vi "KeyboardControl2_PC_Main.vi"() -> ()   [LabVIEW 2014]
uses:
  <vilib>/Utility/inputDevices.llb/keyboardAcquire.vi
  <vilib>/Utility/inputDevices.llb/closeKeyboard.vi
panel:
  in  "Control Selector":bool
  in  "stop":bool
  out "ServoKeyboard":dbl min=-45.0 max=45.0 step=1.0
  out "PropmotorKeybd":dbl min=-9.0 max=9.0 step=1.0
  out "RT Blink":bool
  out "error IO":errorcluster
  out "PC running":bool
  # "Potentiometer"
  # "Use the arrow keys and the \"/\"\nthe change the values"
  # "Keyboard"
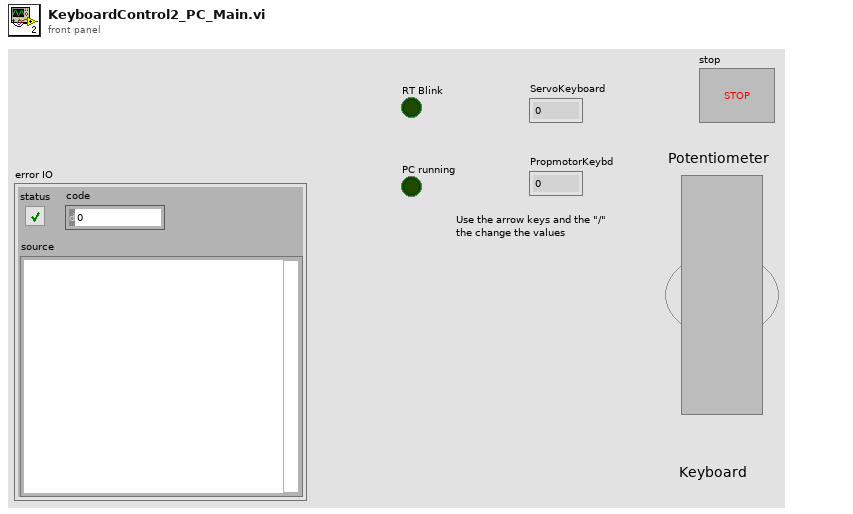
[diagram p1: front panel]
types:
  T1 = enum16{"0", "1", "2", "3", "4", "5", "6", "7", "8", "9", "A", "B", "C", "D", "E", "F", "G", "H", "I", "J", "K", "L", "M", "N", "O", "P", "Q", "R", "S", "T", "U", "V", "W", "X", "Y", "Z", "F1", "F2", "F3", "F4", "F5", "F6", "F7", "F8", "F9", "F10", "F11", "F12", "F13", "F14", "F15", "ADD", "BACK", "BACKSLASH", "CAPITAL", "COMMA", "DECIMAL", "DELETE", "DIVIDE", "DOWN", "END", "EQUALS", "ESCAPE", "GRAVE (`)", "HOME", "INSERT", "LBRACKET", "LCONTROL", "LEFT", "L ALT", "LSHIFT", "LWIN", "MINUS", "MULTIPLY", "NEXT", "NUMLOCK", "NUMPAD_0", "NUMPAD_1", "NUMPAD_2", "NUMPAD_3", "NUMPAD_4", "NUMPAD_5", "NUMPAD_6", "NUMPAD_7", "NUMPAD_8", "NUMPAD_9", "PAUSE", "PERIOD", "PRIOR (PG UP)", "RBRACKET", "RCONTROL", "RETURN", "RIGHT", "R ALT", "RSHIFT", "RWIN", "SCROLL", "SEMICOLON", "SLASH", "SPACE", "SUBTRACT", "TAB", "UP", "ENTER (num pad)", "' (quote)"}[]
  T2 = enum16{"0", "1", "2", "3", "4", "5", "6", "7", "8", "9", "A", "B", "C", "D", "E", "F", "G", "H", "I", "J", "K", "L", "M", "N", "O", "P", "Q", "R", "S", "T", "U", "V", "W", "X", "Y", "Z", "F1", "F2", "F3", "F4", "F5", "F6", "F7", "F8", "F9", "F10", "F11", "F12", "F13", "F14", "F15", "ADD", "BACK", "BACKSLASH", "CAPITAL", "COMMA", "DECIMAL", "DELETE", "DIVIDE", "DOWN", "END", "EQUALS", "ESCAPE", "GRAVE (`)", "HOME", "INSERT", "LBRACKET", "LCONTROL", "LEFT", "L ALT", "LSHIFT", "LWIN", "MINUS", "MULTIPLY", "NEXT", "NUMLOCK", "NUMPAD_0", "NUMPAD_1", "NUMPAD_2", "NUMPAD_3", "NUMPAD_4", "NUMPAD_5", "NUMPAD_6", "NUMPAD_7", "NUMPAD_8", "NUMPAD_9", "PAUSE", "PERIOD", "PRIOR (PG UP)", "RBRACKET", "RCONTROL", "RETURN", "RIGHT", "R ALT", "RSHIFT", "RWIN", "SCROLL", "SEMICOLON", "SLASH", "SPACE", "SUBTRACT", "TAB", "UP", "ENTER (num pad)", "' (quote)"}
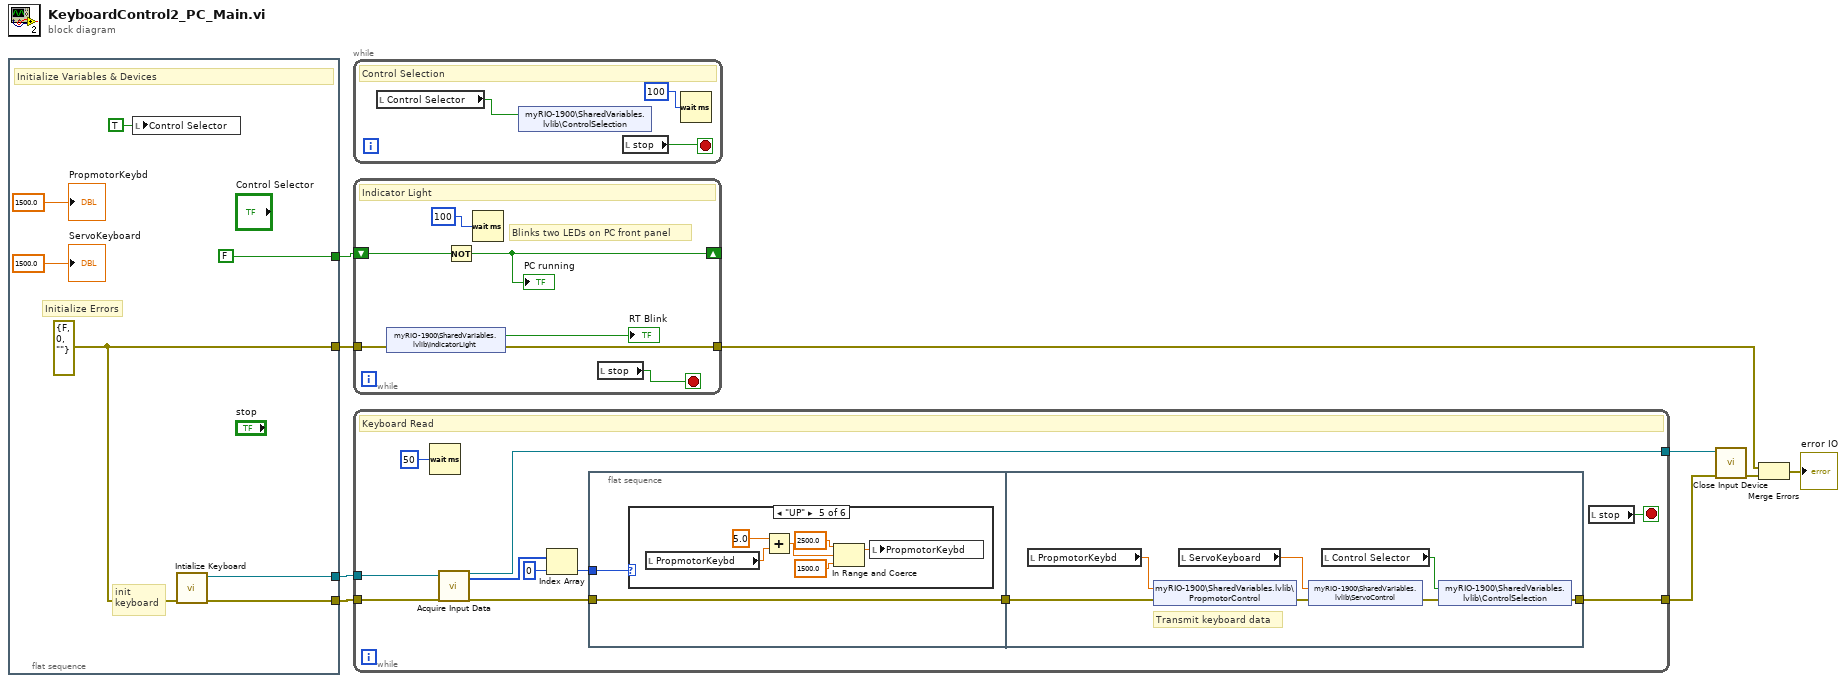
[diagram p0: block diagram]
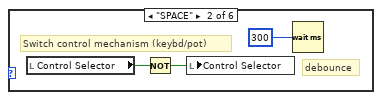
[diagram p3: hidden frame]
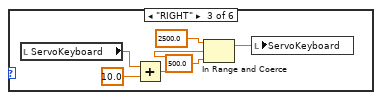
[diagram p4: hidden frame]
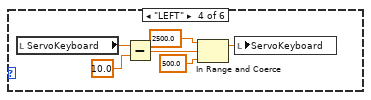
[diagram p5: hidden frame]
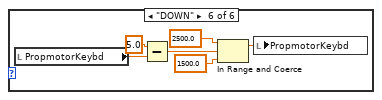
[diagram p6: hidden frame]
diagram:
  n1 = flat-sequence {
    tunnel: [w16] -> w8
    tunnel: [w15] -> w9
    tunnel: [w10] -> w7
    tunnel: [FALSE] -> w4
    frame #0 {
      w10 = errorcluster {"status"=FALSE, "code"=0, "source"=""} ("error in (no error)")
      # "Initialize Errors"
      # "init\nkeyboard"
      # "Initialize Variables & Devices"
      n2 = local write "Control Selector"(TRUE ("Control Selector")) -> ()
      n3 = call <vilib>:"Intialize Keyboard.vi"("error in (no error)"=w10) -> ("error out"=w15:errorcluster, "device ID"=w16:refnum<k1>)  [unwired: 9 in]
      "ServoKeyboard" <- 1500.0 ("ServoKeyboard")
      "PropmotorKeybd" <- 1500.0 ("PropmotorKeybd")
    }
  }
  n4 = while {
    stop <- w19 stop-if-true
    # "Control Selection"
    n5 = local read "Control Selector"() -> (w17:bool)
    n6 = shared-variable "myRIO-1900\\SharedVariables.lvlib\\ControlSelection"(w17) -> ()  [unwired: 1 in, 1 out]
    n7 = local read "stop"() -> (w19:bool)
    n8 = Wait (ms)(milliseconds to wait=u32 100) -> ()  [unwired: 1 out]
  }
  n9 = while {
    shift-right: [w25] -> _
    shift-left: w4 -> [w26]
    tunnel: w7 -> [w24]
    tunnel: [w23] -> w5
    stop <- w20 stop-if-true
    # "Blinks two LEDs on PC front panel"
    # "Indicator Light"
    n10 = shared-variable "myRIO-1900\\SharedVariables.lvlib\\IndicatorLight"(error in=w24) -> (→"RT Blink":bool, error out=w23:errorcluster)
    n11 = Not(x=w26) -> (.not. x?=w25:bool)
    "PC running" <- w25
    n12 = Wait (ms)(milliseconds to wait=u32 100) -> ()  [unwired: 1 out]
    n13 = local read "stop"() -> (w20:bool)
  }
  n14 = while {
    tunnel: w9 -> [w35]
    tunnel: w8 -> [w34]
    tunnel: [w28] -> w3
    tunnel: [w27] -> w2
    stop <- w36 stop-if-true
    # "Keyboard Read"
    n15 = Wait (ms)(milliseconds to wait=u32 50) -> ()  [unwired: 1 out]
    n16 = call-poly <vilib>:"Acquire Input Data.vi"("device ID"=w34, "error in (no error)"=w35) -> ("device ID"=w27:refnum<k1>, "keys pressed"=w33:T1, "error out"=w30:errorcluster)  [unwired: 15 in]
    n17 = Index Array(array=w33, index=0) -> (element=w31:T2)
    n18 = flat-sequence {
      tunnel: w31 -> [w39]
      tunnel: w30 -> [w38]
      tunnel: [w38] -> w29
      tunnel: w29 -> [w72]
      tunnel: [w68] -> w28
      frame #0 {
        n19 = case shown="\"UP\"" w39 {
          frame "0", Default {
          }
          frame "SPACE" {
            # "debounce"
            # "Switch control mechanism (keybd/pot)"
            n20 = local read "Control Selector"() -> (w41:bool)
            n21 = Not(x=w41) -> (.not. x?=w42:bool)
            n22 = local write "Control Selector"(w42) -> ()
            n23 = Wait (ms)(milliseconds to wait=u32 300 ("millisecond timer value")) -> ()  [unwired: 1 out]
          }
          frame "RIGHT" {
            n24 = local read "ServoKeyboard"() -> (w43:dbl)
            n25 = Add(x=w43, y=10.0) -> (x+y=w45:dbl)
            n26 = In Range and Coerce(upper limit=2500.0, x=w45, lower limit=500.0) -> (coerced(x)=w48:dbl)  [unwired: 1 out]
            n27 = local write "ServoKeyboard"(w48) -> ()
          }
          frame "LEFT" {
            n28 = local read "ServoKeyboard"() -> (w50:dbl)
            n29 = Subtract(x=w50, y=10.0) -> (x-y=w51:dbl)
            n30 = In Range and Coerce(upper limit=2500.0, x=w51, lower limit=500.0) -> (coerced(x)=w52:dbl)  [unwired: 1 out]
            n31 = local write "ServoKeyboard"(w52) -> ()
          }
          frame "UP" {
            n32 = local read "PropmotorKeybd"() -> (w55:dbl)
            n33 = Add(x=5.0, y=w55) -> (x+y=w58:dbl)
            n34 = In Range and Coerce(upper limit=2500.0, x=w58, lower limit=1500.0) -> (coerced(x)=w59:dbl)  [unwired: 1 out]
            n35 = local write "PropmotorKeybd"(w59) -> ()
          }
          frame "DOWN" {
            n36 = local read "PropmotorKeybd"() -> (w66:dbl)
            n37 = Subtract(x=5.0, y=w66) -> (x-y=w63:dbl)
            n38 = In Range and Coerce(upper limit=2500.0, x=w63, lower limit=1500.0) -> (coerced(x)=w62:dbl)  [unwired: 1 out]
            n39 = local write "PropmotorKeybd"(w62) -> ()
          }
        }
      }
      frame #1 {
        # "Transmit keyboard data"
        n40 = local read "PropmotorKeybd"() -> (w73:dbl)
        n41 = shared-variable "myRIO-1900\\SharedVariables.lvlib\\PropmotorControl"(w73, error in=w72) -> (error out=w71:errorcluster)
        n42 = local read "ServoKeyboard"() -> (w70:dbl)
        n43 = shared-variable "myRIO-1900\\SharedVariables.lvlib\\ServoControl"(w70, error in=w71) -> (error out=w67:errorcluster)
        n44 = local read "Control Selector"() -> (w69:bool)
        n45 = shared-variable "myRIO-1900\\SharedVariables.lvlib\\ControlSelection"(w69, error in=w67) -> (error out=w68:errorcluster)
      }
    }
    n46 = local read "stop"() -> (w36:bool)
  }
  n47 = call-poly <vilib>:"Close Input Device.vi"("error in (no error)"=w3, "device ID"=w2) -> ("error out"=w1:errorcluster)  [unwired: 8 in]
  n48 = Merge Errors(w5, w1) -> (→"error IO":errorcluster)
